vi "Periodic Tasks.vi"(8 "error in (no error)":errorcluster, 10 "Co_fifo":refnum<k33>, 11 "Drive Fifo":refnum<k33>) -> ()   [LabVIEW 2014]
doc: "This VI runs in parallel to other tasks. It can contain as many user-defined periodic loops as you need. These can carry out PID or other sorts of timed response."
uses:
  Lightning base/TeleopCmd.ctl
  Lightning base/CmdFlag.ctl
  Lightning base/Co-Pilot_game_control.ctl
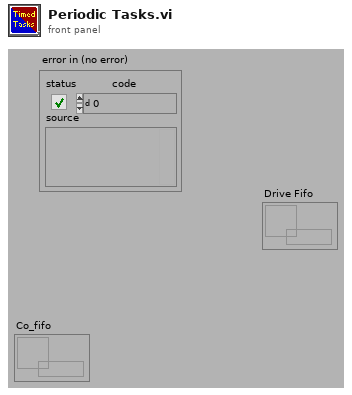
[diagram p1: front panel]
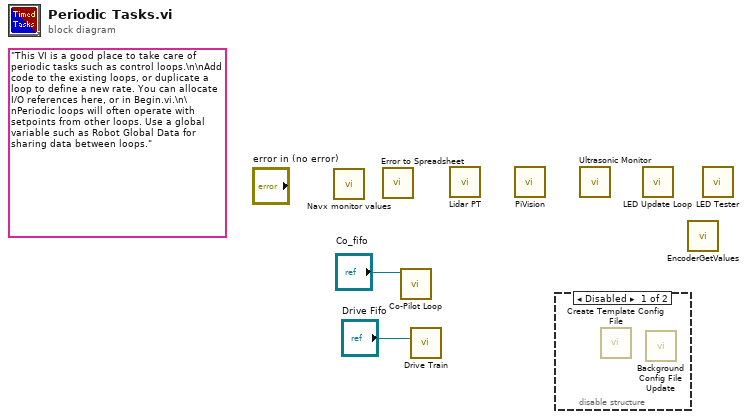
[diagram p0: block diagram]
diagram:
  (unwired) "This VI is a good place to take care of periodic tasks such as control loops.\n\nAdd code to the existing loops, or duplicate a loop to define a new rate. You can allocate I/O references here, or in Begin.vi.\n\nPeriodic loops will often operate with setpoints from other loops. Use a global variable such as Robot Global Data for sharing data between loops."
  n1 = call "Navx monitor values.vi"() -> ()  [unwired: 12 in]
  n2 = call "Error to Spreadsheet.vi"() -> ()  [unwired: 12 in]
  n3 = call "Co-Pilot Loop.vi"("Co_fifo"="Co_fifo") -> ()  [unwired: 11 in]
  n4 = call "Drive Train.vi"("Refnum in"="Drive Fifo") -> ()  [unwired: 11 in]
  n5 = call "Lidar PT.vi"() -> ()  [unwired: 12 in]
  n6 = call "PiVision.vi"() -> ()  [unwired: 12 in]
  n7 = disable-structure shown="Disabled" {
    frame Disabled {
      n8 = call "Create Template Config File.vi"() -> ()  [unwired: 11 in, 1 out]
      n9 = call "Background Config File Update.vi"() -> ()  [unwired: 12 in]
    }
    frame Enabled {
    }
  }
  n10 = call "Ultrasonic Monitor.vi"() -> ()  [unwired: 12 in]
  n11 = call "LED Update Loop.vi"() -> ()  [unwired: 12 in]
  n12 = call "EncoderGetValues.vi"() -> ()  [unwired: 12 in]
  n13 = call "LED Tester.vi"() -> ()  [unwired: 12 in]
